vi "IOPanel_HandShake.vi"(11 "IOCard In":refnum<class "IOCard.lvclass">) -> ()   [LabVIEW 2019]
uses:
  Ctrl/IO Card_Type.ctl
  IO_Class/IOCard.lvclass
  <vilib>/Utility/miscctls.llb/LVPositionTypeDef.ctl
  IO_Class/IOCard.lvclass/IOCard.ctl
  LLB/Message/Ctrl/MsgDataInput.ctl
  LLB/Message/Ctrl/MsgPageSelect.ctl
  LLB/Message/Ctrl/LogType.ctl
  IO_Class/6480/6480.lvclass
  C:/Users/MyUser/Desktop/204J1_20201007/System/Function/IO Folder/IO_Class/IOCard.lvclass
  IO_Class/2410C/2410C-64.lvclass
  IO_Class/Zan/ZanCard.lvclass
  IO_Class/DMC1000B/DMC1000B.lvclass
  IO_Class/16InOut/16InOut.lvclass
  global/InAndOutGB.vi
  LLB/Commonly VI/Main Glb.vi
  <vilib>/Utility/config.llb/Read Key (String).vi
  LLB/Commonly VI.lvlib
  <vilib>/Utility/config.llb/NI_LVConfig.lvlib
  LLB/Message/MsgShowAndLog.lvlib
panel:
  out "IOCard":refnum<class "IOCard.lvclass">
  out "Card_Type":T1
  out "QName":string
  in  "Tab Control":enum32{"Input", "Output"}(tab)
  in  "Reconnect":bool
  out "Lst_Input":i32[](listbox) caption="Input"
  in  "Lst_Output":i32[](listbox)=[2] caption="Output"
  out "CardNumber":i32
  out "IOType":enum16{"Input", "Output"}(ring)=enum."Output"
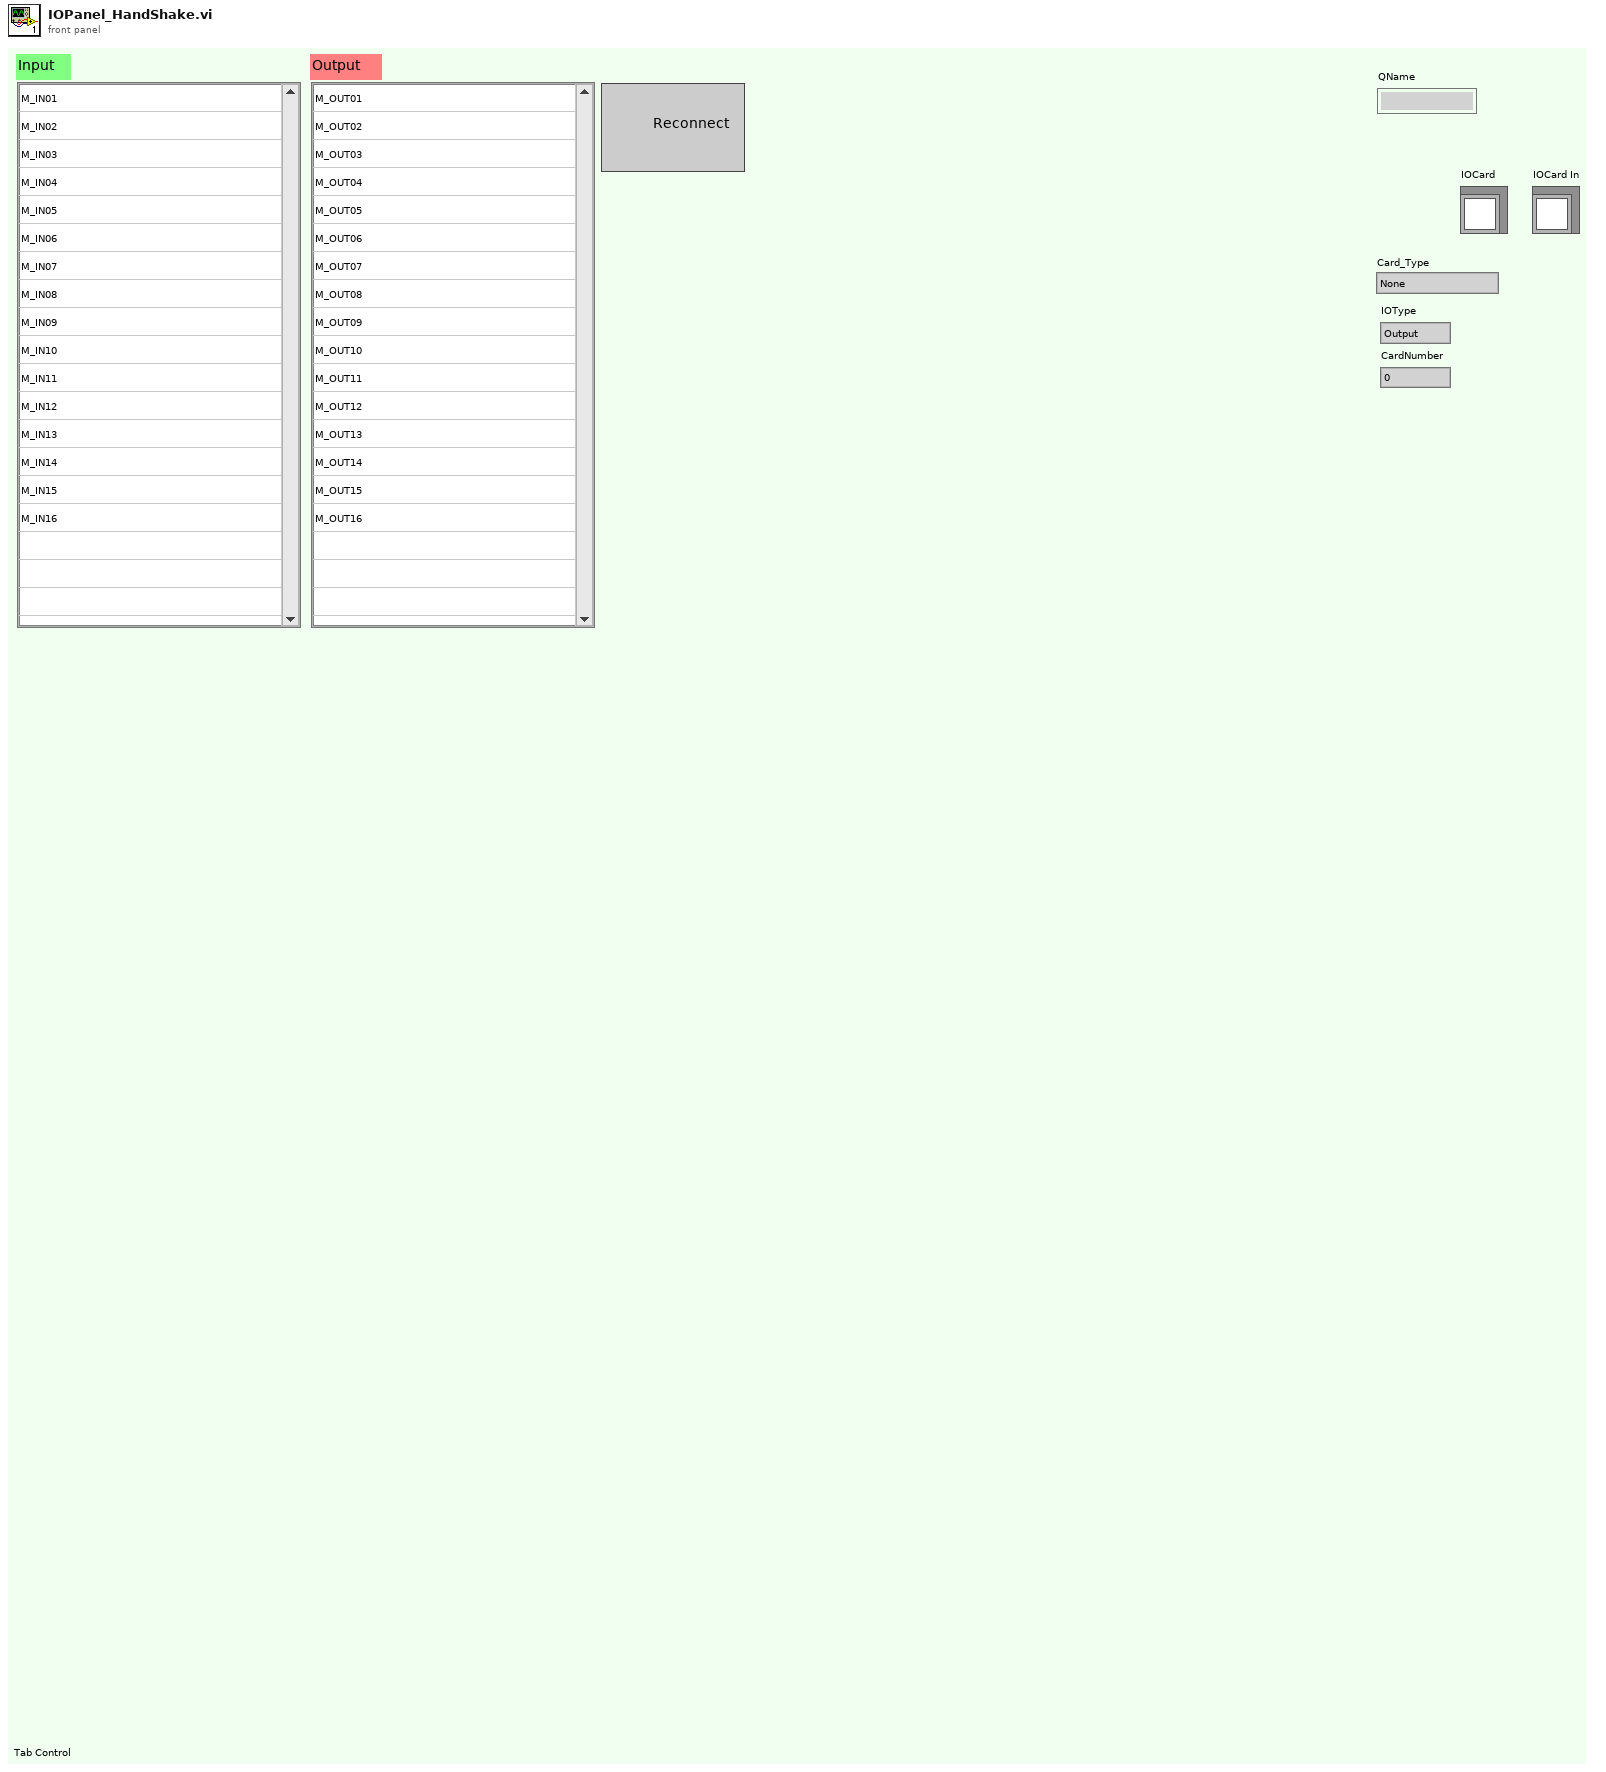
[diagram p1: front panel]
types:
  T1 = typedef "IO Card_Type.ctl" = enum16{"None", "Unidaq32", "6480", "2410C-64", "Zan", "DMC1000B", "16InOut", "Robot", "DMC3600"}
  T2 = typedef "LVPositionTypeDef.ctl" = cluster{"Left":i32, "Top":i32}
  T3 = cluster{"IO Card Type":T1, "IOType":enum16{"Input", "Output"}, "CardNumber":i32, "ConnectAct":bool, "IP":string}
  T4 = cluster{"CardNumber":i32, "Connect":bool, "Handler":i32}
  T5 = typedef "MsgDataInput.ctl" = cluster{"MsgPageSelect":T6, "LogType":T7, "Msg":string, "Time":string}
  T6 = typedef "MsgShowAndLog.lvlib/MsgPageSelect.ctl" = enum16{"System", "Comm", "IO", "Action", "Alarm"}
  T7 = typedef "MsgShowAndLog.lvlib/LogType.ctl" = enum16{"Auto", "Manual", "Handshake", "Error"}
  T8 = typedef "LVBoundsTypeDef.ctl" = cluster{"Width":u32, "Height":u32}
  T9 = typedef "LVPoint32TypeDef.ctl" = cluster{"Horizontal":i32, "Vertical":i32}
  T10 = typedef "NI_LVConfig.lvlib/Config Data RefNum.ctl" = refnum<k1>
  T11 = cluster{"Card":i32, "Connect":bool, "Handler":i32}[]
  T12 = cluster{"Card":i32, "Connect":bool, "Handler":i32}
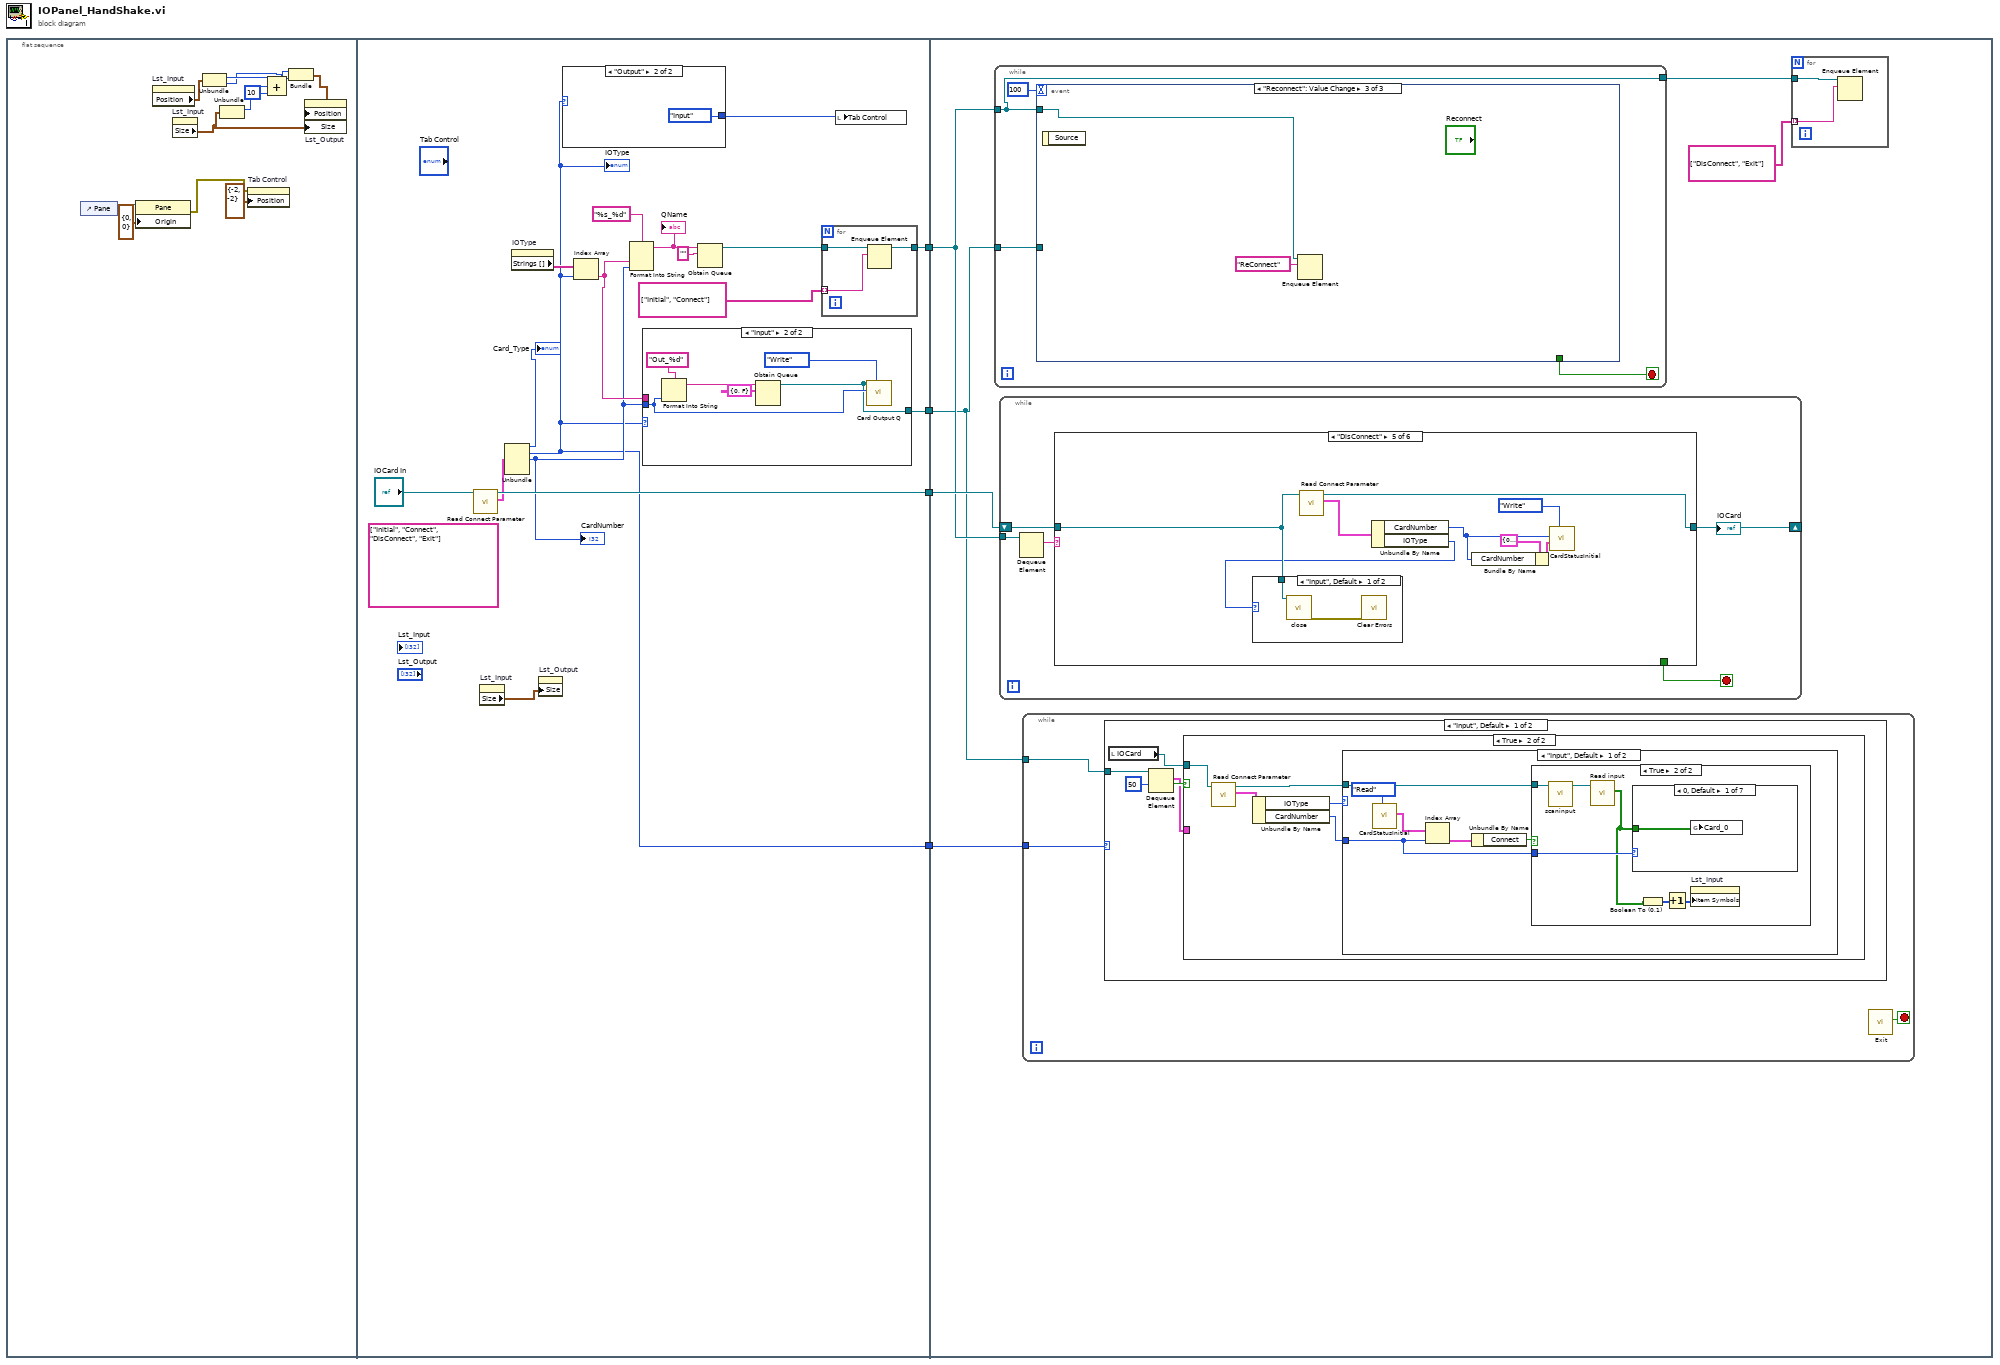
[diagram p0: block diagram]
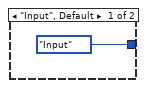
[diagram p2: hidden frame]
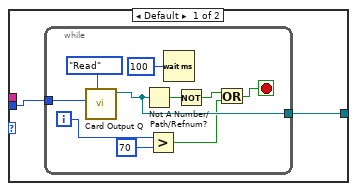
[diagram p3: hidden frame]
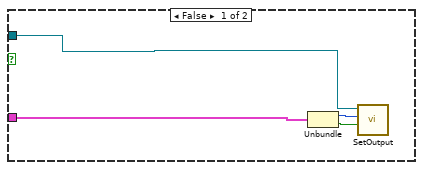
[diagram p4: hidden frame]
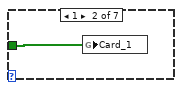
[diagram p6: hidden frame]
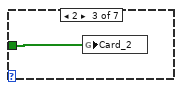
[diagram p7: hidden frame]
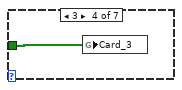
[diagram p8: hidden frame]
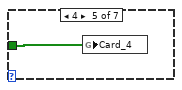
[diagram p9: hidden frame]
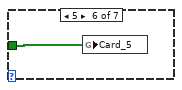
[diagram p10: hidden frame]
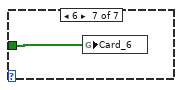
[diagram p11: hidden frame]
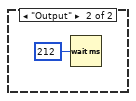
[diagram p13: hidden frame]
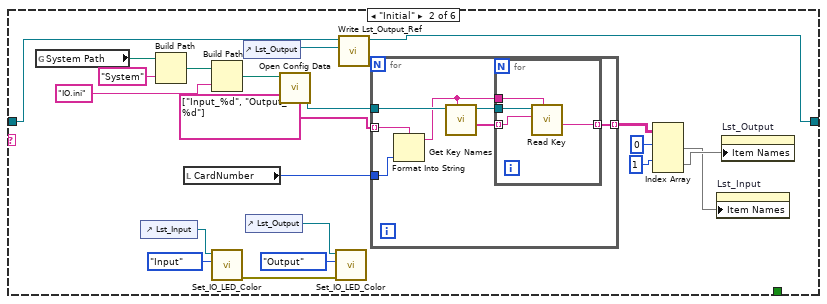
[diagram p15: hidden frame]
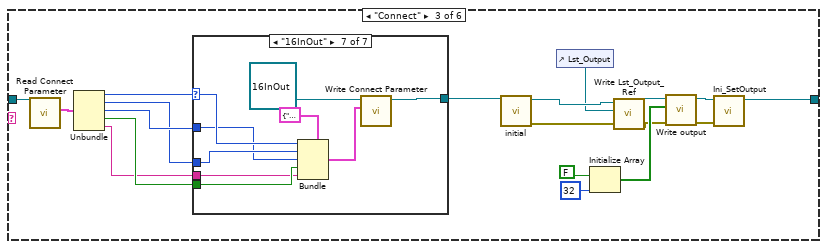
[diagram p16: hidden frame]
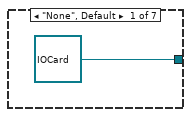
[diagram p17: hidden frame]
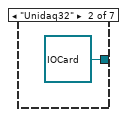
[diagram p18: hidden frame]
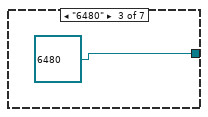
[diagram p19: hidden frame]
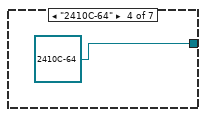
[diagram p20: hidden frame]
diagram:
  n1 = flat-sequence {
    tunnel: [w30] -> w4
    tunnel: [w25] -> w3
    tunnel: [w23] -> w2
    tunnel: [w17] -> w1
    tunnel: w4 -> [w62]
    tunnel: w3 -> [w59]
    tunnel: w2 -> [w58]
    tunnel: w1 -> [w57]
    frame #0 {
      n2 = control-ref of="Pane"() -> (w15:refnum<vi>)
      n3 = property class="Pane"(reference=w15, "Origin"=T2 {"Left"=0, "Top"=0} ("Position")) -> (error out=w13:errorcluster)  [unwired: 1 in, 1 out]
      n4 = property on="Lst_Input" class="LstBox (strict)"() -> ("Position"=w12:T2)  [unwired: 2 in, 2 out]
      n5 = property on="Lst_Input" class="LstBox (strict)"() -> ("Size"=w11:T8)  [unwired: 2 in, 2 out]
      n6 = Unbundle(w12) -> ("Left"=w10:i32, "Top"=w6:i32)
      n7 = Unbundle(w11) -> ("Width"=w9:u32)  [unwired: 1 out]
      n8 = property on="Tab Control" class="TabCtl (strict)"(error in=w13, "Position"=T2 {"Left"=-2, "Top"=-2}) -> ()  [unwired: 1 in, 2 out]
      n9 = Compound Arithmetic op=ADD(w10, w9, u32 10 ("value")) -> (w7:u32)
      n10 = Bundle(w7, "Top"=w6) -> (w5:cluster{u32, "Top":i32})  [unwired: 1 in]
      n11 = property on="Lst_Output" class="LstBox (strict)"("Position"=w5, "Size"=w11) -> ()  [unwired: 2 in, 2 out]
    }
    frame #1 {
      (unwired) string[] ["Initial", "Connect", "DisConnect", "Exit"]
      n12 = call "Read Connect Parameter.vi"("IOCard in"="IOCard In") -> ("Connect Parameter"=w29:T3, "IOCard out"=w30:refnum<class "IOCard.lvclass">)  [unwired: 8 in, 1 out]
      n13 = property on="Lst_Input" class="LstBox (strict)"() -> ("Size"=w18:T8)  [unwired: 2 in, 2 out]
      n14 = Unbundle(w29) -> ("IO Card Type"=→"Card_Type":T1, "IOType"=w17:enum16{"Input", "Output"}, "CardNumber"=w21:i32)  [unwired: 2 out]
      "CardNumber" <- w21
      "IOType" <- w17
      n15 = property on="IOType" class="Enum (strict)"() -> ("Strings []"=w28:string[])  [unwired: 2 in, 2 out]
      n16 = property on="Lst_Output" class="LstBox (strict)"("Size"=w18) -> ()  [unwired: 2 in, 2 out]
      n17 = case shown="\"Output\"" w17 {
        tunnel: [enum32{"Input", "Output"}."Input" ("Tab Control") enum32{"Input", "Output"}."Input" ("Tab Control")] -> w19
        frame "Input", Default {
        }
        frame "Output" {
        }
      }
      n18 = Index Array(array=w28, index=w17) -> (element=w24:string)
      n19 = Format Into String(format string="%s_%d", w24, w21) -> (resulting string=w32:string)  [unwired: 2 in, 1 out]
      "QName" <- w32
      n20 = case shown="\"Input\"" w17 {
        tunnel: w24 -> [_ _]
        tunnel: w21 -> [w37 w50]
        tunnel: [w36 w49] -> w23
        frame Default {
          n21 = while {
            tunnel: w37 -> [w46]
            tunnel: [w44] -> w36
            i -> [w40]
            stop <- w43 stop-if-true
            n22 = call "Card Output Q.vi"("Action"=enum16{"Initial", "Write", "Read", "Release"}."Read", "CardIndex"=w46) -> ("Output Q Out"=w44:refnum<queue>)  [unwired: 8 in, 1 out]
            n23 = Not A Number/Path/Refnum?(number/path/refnum=w44) -> (NaN/Path/Refnum?=w42:bool)
            n24 = Greater?(x=w40, y=70) -> (0:w39:bool)
            n25 = Wait (ms)(milliseconds to wait=u32 100) -> ()  [unwired: 1 out]
            n26 = Not(x=w42) -> (.not. x?=w41:bool)
            n27 = Or(x=w41, y=w39) -> (x .or. y?=w43:bool)
          }
        }
        frame "Input" {
          n28 = Format Into String(format string="Out_%d", w50) -> (resulting string=w48:string)  [unwired: 2 in, 1 out]
          n29 = Obtain Queue(name (unnamed)=w48, element data type=cluster{"Index":i32, "BL":bool} {"Index"=0, "BL"=FALSE}) -> (queue out=w49:refnum<queue>)  [unwired: 3 in, 2 out]
          n30 = call "Card Output Q.vi"("Action"=enum16{"Initial", "Write", "Read", "Release"}."Write", "CardIndex"=w50, "OutputQIn"=w49) -> ()  [unwired: 7 in, 2 out]
        }
      }
      n31 = Obtain Queue(name (unnamed)=w32, element data type="") -> (queue out=w26:refnum<queue>)  [unwired: 3 in, 2 out]
      n32 = for {
        tunnel: w26 -> [w56]
        tunnel: string[] ["Initial", "Connect"] -> [w55] mode=indexing
        tunnel: [w54] -> w25
        n33 = Enqueue Element(queue=w56, element=w55) -> (queue out=w54:refnum<queue>)  [unwired: 2 in, 2 out]
      }
      n34 = local write "Tab Control"(w19) -> ()
    }
    frame #2 {
      n35 = while {
        tunnel: w59 -> [w246]
        tunnel: [w246] -> w61
        tunnel: w58 -> [w245]
        stop <- w247 stop-if-true
        n36 = event shown="[2] \"Reconnect\": Value Change" {
          selector: _ -> [_ _ _]
          dyn-events: _ -> [_ _ _]
          timeout: 100 -> [_ _ _]
          tunnel: [w249 _ _] -> w247
          tunnel: w246 -> [_ _ w268]
          tunnel: w245 -> [_ w261 _]
          event Timeout {
            n37 = event-data() -> ()  [unwired: 1 in, 3 out]
            n38 = call "Exit.vi"() -> ("ExitOut"=w249:bool)  [unwired: 11 in]
          }
          event "Lst_Output": Double Click {
            n39 = event-data() -> ("CtlRef"=w266:refnum<vi>, "Coords"=w265:T9)  [unwired: 1 in, 1 out]
            n40 = invoke on="Invoke Node" class="LstBox (strict)" method="Point To Row"(reference=w266, "Point"=w265) -> (reference out=w262:refnum<vi>, "Row"=w253:i32)  [unwired: 5 in, 5 out]
            n41 = property on="Property Node" class="LstBox (strict)"(reference=w262) -> ("Item Symbols"=w250:i32[])  [unwired: 1 in, 2 out]
            n42 = Index Array(array=w250, index=w253) -> (element=w264:i32)
            n43 = Equal?(x=w264, y=1) -> (x = y?=w252:bool)
            n44 = Bundle(cluster=cluster{"Index":i32, "BL":bool} {"Index"=0, "BL"=FALSE} ("element"), "Index"=w253, "BL"=w252) -> (w260:cluster{"Index":i32, "BL":bool})
            n45 = local read "QName"() -> (w254:string)
            n46 = Enqueue Element(queue=w261, element=w260) -> (error out=w251:errorcluster)  [unwired: 2 in, 2 out]
            n47 = Format Into String(format string="%s,%d,%s", w254, w253, w252) -> (resulting string=w256:string)  [unwired: 2 in, 1 out]
            n48 = Bundle By Name(cluster=T5 {"MsgPageSelect"=enum."IO", "LogType"=enum."Manual", "Msg"="", "Time"=""} ("DataIn"), "Msg"=w256) -> (w258:T5)
            n49 = call "SendMsg.vi"("error in (no error)"=w251, "DataIn"=w258) -> ()  [unwired: 9 in, 1 out]
          }
          event "Reconnect": Value Change {
            n50 = event-data() -> ()  [unwired: 1 in, 1 out]
            n51 = Enqueue Element(queue=w268, element="ReConnect") -> ()  [unwired: 2 in, 3 out]
          }
        }
      }
      n52 = while {
        tunnel: w59 -> [w106]
        shift-right: [w104] -> _
        shift-left: w62 -> [w103]
        stop <- w102 stop-if-true
        n53 = Dequeue Element(queue=w106) -> (element=w105:string)  [unwired: 2 in, 3 out]
        n54 = case shown="\"DisConnect\"" w105 {
          tunnel: [w107 w116 w153 w194 w234 w243] -> w104
          tunnel: w103 -> [w107 w117 w158 w199 w235 w243]
          tunnel: [_ _ _ _ _ TRUE] -> w102
          frame "False", Default {
          }
          frame "Initial" {
            n55 = global read "Main Glb.vi" "System Path"() -> (w128:path)
            n56 = control-ref of="Lst_Input"() -> (w121:refnum<vi>)
            n57 = Build Path(base path=w128, name or relative path="System") -> (appended path=w126:path)
            n58 = local read "CardNumber"() -> (w108:i32)
            n59 = Build Path(base path=w126, name or relative path="IO.ini") -> (appended path=w124:path)
            n60 = call "Set_IO_LED_Color.vi"("SelectType"=enum16{"Input", "Output"}."Input", "ListBox Ref"=w121) -> ("error out"=w118:errorcluster)  [unwired: 9 in]
            n61 = control-ref of="Lst_Output"() -> (w115:refnum<vi>)
            n62 = control-ref of="Lst_Output"() -> (w122:refnum<vi>)
            n63 = call <vilib>:"Open Config Data.vi"("configuration file path"=w124) -> ("refnum"=w123:T10)  [unwired: 8 in, 2 out]
            n64 = call "Set_IO_LED_Color.vi"("error in (no error)"=w118, "SelectType"=enum16{"Input", "Output"}."Output", "ListBox Ref"=w122) -> ()  [unwired: 8 in, 1 out]
            n65 = call-dynamic "Write Lst_Output_Ref.vi"("Lst_Output_Ref"=w115, "IOCard in"=w117) -> ("IOCard out"=w116:refnum<class "IOCard.lvclass">)  [unwired: 8 in, 1 out]
            n66 = for {
              tunnel: w123 -> [w135]
              tunnel: [w132] -> w113 mode=indexing
              tunnel: string[] ["Input_%d", "Output_%d"] -> [w131] mode=indexing
              tunnel: w108 -> [w129]
              n67 = Format Into String(format string=w131, w129) -> (resulting string=w130:string)  [unwired: 2 in, 1 out]
              n68 = call <vilib>:"Get Key Names.vi"("section"=w130, "refnum"=w135) -> ("key names"=w133:string[], "refnum out"=w134:T10)  [unwired: 6 in, 2 out]
              n69 = for {
                tunnel: w134 -> [w139]
                tunnel: w133 -> [w138] mode=indexing
                tunnel: w130 -> [w137]
                tunnel: [w136] -> w132 mode=indexing
                n70 = call-poly <vilib>:"Read Key.vi"("section"=w137, "key"=w138, "refnum"=w139) -> ("value"=w136:string)  [unwired: 5 in, 3 out]
              }
            }
            n71 = Index Array(array=w113, index (row) #1=0 ("index (row)"), index (row) #2=1 ("index (row)")) -> (element #1=w109:string[], element #2=w110:string[])  [unwired: 2 in]
            n72 = property on="Lst_Input" class="LstBox (strict)"("Item Names"=w109) -> ()  [unwired: 2 in, 2 out]
            n73 = property on="Lst_Output" class="LstBox (strict)"("Item Names"=w110) -> ()  [unwired: 2 in, 2 out]
          }
          frame "Connect" {
            n74 = call "Read Connect Parameter.vi"("IOCard in"=w158) -> ("Connect Parameter"=w157:T3)  [unwired: 8 in, 2 out]
            n75 = Unbundle(w157) -> ("IO Card Type"=w156:T1, "IOType"=w154:enum16{"Input", "Output"}, "CardNumber"=w155:i32, "ConnectAct"=w151:bool, "IP"=w150:string)
            n76 = case shown="\"16InOut\"" w156 {
              selector: w156 -> [_ _ _ _ _ w169 w178]
              tunnel: [refnum<class "IOCard.lvclass"> refnum ("IOCard.lvclass") refnum<class "IOCard.lvclass"> refnum ("IOCard.lvclass") refnum<class "6480.lvclass"> refnum ("6480.lvclass") refnum<class "2410C-64.lvclass"> refnum ("2410C-64.lvclass") refnum<class "ZanCard.lvclass"> refnum ("ZanCard.lvclass") w172 w181] -> w149
              tunnel: w155 -> [_ _ _ _ _ w167 w176]
              tunnel: w154 -> [_ _ _ _ _ w168 w177]
              tunnel: w151 -> [_ _ _ _ _ w166 w175]
              tunnel: w150 -> [_ _ _ _ _ w165 w174]
              frame "None", Default {
              }
              frame "Unidaq32" {
              }
              frame "6480" {
              }
              frame "2410C-64" {
              }
              frame "Zan" {
              }
              frame "DMC1000B" {
                w164 = refnum<class "DMC1000B.lvclass"> refnum  # DMC1000B.lvclass
                n77 = Bundle(cluster=T3 {"IO Card Type"=enum."None", "IOType"=enum."Output", "CardNumber"=0, "ConnectAct"=FALSE, "IP"=""} ("Connect Parameter"), "IO Card Type"=w169, "IOType"=w168, "CardNumber"=w167, "ConnectAct"=w166, "IP"=w165) -> (w170:T3)
                n78 = call "Write Connect Parameter.vi"("Connect Parameter"=w170, "IOCard in"=w164) -> ("IOCard out"=w172:refnum<class "DMC1000B.lvclass">)  [unwired: 8 in, 1 out]
              }
              frame "16InOut" {
                n79 = Bundle(cluster=T3 {"IO Card Type"=enum."None", "IOType"=enum."Output", "CardNumber"=0, "ConnectAct"=FALSE, "IP"=""} ("Connect Parameter"), "IO Card Type"=w178, "IOType"=w177, "CardNumber"=w176, "ConnectAct"=w175, "IP"=w174) -> (w179:T3)
                n80 = call "Write Connect Parameter.vi"("Connect Parameter"=w179, "IOCard in"=refnum<class "16InOut.lvclass"> refnum ("16InOut.lvclass")) -> ("IOCard out"=w181:refnum<class "16InOut.lvclass">)  [unwired: 8 in, 1 out]
              }
            }
            n81 = call-dynamic "initial.vi"("IOCard in"=w149) -> ("error out"=w141:errorcluster, "IOCard out"=w152:refnum<class "IOCard.lvclass">)  [unwired: 9 in]
            n82 = control-ref of="Lst_Output"() -> (w142:refnum<vi>)
            n83 = Initialize Array(FALSE, 32 ("dimension size")) -> (w147:bool[])
            n84 = call-dynamic "Write Lst_Output_Ref.vi"("error in (no error)"=w141, "Lst_Output_Ref"=w142, "IOCard in"=w152) -> ("error out"=w144:errorcluster, "IOCard out"=w143:refnum<class "IOCard.lvclass">)  [unwired: 7 in]
            n85 = call-dynamic "Write output.vi"("error in (no error)"=w144, "output"=w147, "IOCard in"=w143) -> ("error out"=w140:errorcluster, "IOCard out"=w148:refnum<class "IOCard.lvclass">)  [unwired: 7 in]
            n86 = call-dynamic "Ini_SetOutput.vi"("error in (no error)"=w140, "IOCard in"=w148) -> ("IOCard out"=w153:refnum<class "IOCard.lvclass">)  [unwired: 8 in, 1 out]
          }
          frame "ReConnect" {
            n87 = call "Read Connect Parameter.vi"("IOCard in"=w199) -> ("Connect Parameter"=w198:T3)  [unwired: 8 in, 2 out]
            n88 = Unbundle(w198) -> ("IO Card Type"=w197:T1, "IOType"=w195:enum16{"Input", "Output"}, "CardNumber"=w196:i32, "ConnectAct"=w192:bool, "IP"=w191:string)
            n89 = case shown="\"16InOut\"" w197 {
              selector: w197 -> [_ _ _ _ _ w217 w229]
              tunnel: [refnum<class "IOCard.lvclass"> refnum ("IOCard.lvclass") refnum<class "IOCard.lvclass"> refnum ("IOCard.lvclass") refnum<class "6480.lvclass"> refnum ("6480.lvclass") refnum<class "2410C-64.lvclass"> refnum ("2410C-64.lvclass") refnum<class "ZanCard.lvclass"> refnum ("ZanCard.lvclass") w220 w232] -> w190
              tunnel: w196 -> [_ _ _ _ _ w215 w227]
              tunnel: w195 -> [_ _ _ _ _ w216 w228]
              tunnel: w192 -> [_ _ _ _ _ w214 w226]
              tunnel: w191 -> [_ _ _ _ _ w213 _]
              tunnel: "$VISA resource name" ("element") -> [_ _ _ _ _ _ w221]
              frame "None", Default {
              }
              frame "Unidaq32" {
              }
              frame "6480" {
              }
              frame "2410C-64" {
              }
              frame "Zan" {
              }
              frame "DMC1000B" {
                w212 = refnum<class "DMC1000B.lvclass"> refnum  # DMC1000B.lvclass
                n90 = Bundle(cluster=T3 {"IO Card Type"=enum."None", "IOType"=enum."Output", "CardNumber"=0, "ConnectAct"=FALSE, "IP"=""} ("Connect Parameter"), "IO Card Type"=w217, "IOType"=w216, "CardNumber"=w215, "ConnectAct"=w214, "IP"=w213) -> (w218:T3)
                n91 = call "Write Connect Parameter.vi"("Connect Parameter"=w218, "IOCard in"=w212) -> ("IOCard out"=w220:refnum<class "DMC1000B.lvclass">)  [unwired: 8 in, 1 out]
              }
              frame "16InOut" {
                n92 = call "SystemSearchDataName.vi"("element"=w221) -> ("variant"=w224:variant)  [unwired: 8 in, 2 out]
                n93 = Variant To Data(type=refnum<visa-resource-name> refnum ("VISA resource name"), Variant=w224) -> (data=w222:refnum<visa-resource-name>)  [unwired: 1 in, 1 out]
                n94 = Bundle(cluster=T3 {"IO Card Type"=enum."None", "IOType"=enum."Output", "CardNumber"=0, "ConnectAct"=FALSE, "IP"=""} ("Connect Parameter"), "IO Card Type"=w229, "IOType"=w228, "CardNumber"=w227, "ConnectAct"=w226, "IP"=w222) -> (w230:T3)
                n95 = call "Write Connect Parameter.vi"("Connect Parameter"=w230, "IOCard in"=refnum<class "16InOut.lvclass"> refnum ("16InOut.lvclass")) -> ("IOCard out"=w232:refnum<class "16InOut.lvclass">)  [unwired: 8 in, 1 out]
              }
            }
            n96 = call-dynamic "initial.vi"("IOCard in"=w190) -> ("error out"=w183:errorcluster, "IOCard out"=w193:refnum<class "IOCard.lvclass">)  [unwired: 9 in]
            n97 = control-ref of="Lst_Output"() -> (w184:refnum<vi>)
            n98 = Initialize Array(FALSE, 32 ("dimension size")) -> (w189:bool[])
            n99 = call-dynamic "Write Lst_Output_Ref.vi"("error in (no error)"=w183, "Lst_Output_Ref"=w184, "IOCard in"=w193) -> ("error out"=w186:errorcluster, "IOCard out"=w185:refnum<class "IOCard.lvclass">)  [unwired: 7 in]
            n100 = disable-structure shown="Enabled" {
              disable-tunnel: [w205 w206] -> w194
              disable-tunnel: w189 -> [w203 _]
              disable-tunnel: w186 -> [w202 _]
              disable-tunnel: w185 -> [w201 w206]
              frame Disabled {
                n101 = call-dynamic "Write output.vi"("error in (no error)"=w202, "output"=w203, "IOCard in"=w201) -> ("error out"=w200:errorcluster, "IOCard out"=w204:refnum<class "IOCard.lvclass">)  [unwired: 7 in]
                n102 = call-dynamic "Ini_SetOutput.vi"("error in (no error)"=w200, "IOCard in"=w204) -> ("IOCard out"=w205:refnum<class "IOCard.lvclass">)  [unwired: 8 in, 1 out]
              }
              frame Enabled {
              }
            }
          }
          frame "DisConnect" {
            n103 = call "Read Connect Parameter.vi"("IOCard in"=w235) -> ("Connect Parameter"=w239:T3, "IOCard out"=w234:refnum<class "IOCard.lvclass">)  [unwired: 8 in, 1 out]
            n104 = Unbundle By Name(w239) -> ("CardNumber"=w236:i32, "IOType"=w233:enum16{"Input", "Output"})
            n105 = case shown="\"Input\", Default" w233 {
              tunnel: w235 -> [w241 _]
              frame "Input", Default {
                n106 = call-dynamic "close.vi"("IOCard in"=w241) -> ("error out"=w242:errorcluster)  [unwired: 9 in, 1 out]
                n107 = call <vilib>:"Clear Errors.vi"("error in (no error)"=w242) -> ()  [unwired: 5 in, 2 out]
              }
              frame "Output" {
              }
            }
            n108 = Bundle By Name(cluster=T4 {"CardNumber"=0, "Connect"=FALSE, "Handler"=0} ("DataIn"), "CardNumber"=w236) -> (w237:T4)
            n109 = call "CardStatusInitial.vi"("Action"=enum16{"Initial", "Write", "Read", "Release"}."Write", "DataIn"=w237, "CardNumber"=w236) -> ()  [unwired: 8 in, 1 out]
          }
          frame "Exit" {
          }
        }
        "IOCard" <- w104
      }
      n110 = while {
        tunnel: w58 -> [w64]
        tunnel: w57 -> [w63]
        stop <- w65 stop-if-true
        n111 = case shown="\"Input\", Default" w63 {
          tunnel: w64 -> [w70 _]
          frame "Input", Default {
            n112 = local read "IOCard"() -> (w66:refnum<class "IOCard.lvclass">)
            n113 = Dequeue Element(queue=w70, timeout in ms (-1)=50) -> (element=w67:cluster{"Index":i32, "BL":bool}, timed out?=w68:bool)  [unwired: 1 in, 2 out]
            n114 = case shown="True" w68 {
              tunnel: w67 -> [w74 _]
              tunnel: w66 -> [w71 w77]
              frame False {
                n115 = Unbundle(w74) -> ("Index"=w73:i32, "BL"=w72:bool)
                n116 = call-dynamic "SetOutput.vi"("Boolean"=w72, "Index"=w73, "IOCard in"=w71) -> ()  [unwired: 6 in, 3 out]
              }
              frame True {
                n117 = call "Read Connect Parameter.vi"("IOCard in"=w77) -> ("Connect Parameter"=w76:T3, "IOCard out"=w78:refnum<class "IOCard.lvclass">)  [unwired: 8 in, 1 out]
                n118 = Unbundle By Name(w76) -> ("IOType"=w75:enum16{"Input", "Output"}, "CardNumber"=w79:i32)
                n119 = case shown="\"Input\", Default" w75 {
                  tunnel: w78 -> [w85 _]
                  tunnel: w79 -> [w80 _]
                  frame "Input", Default {
                    n120 = call "CardStatusInitial.vi"("Action"=enum16{"Initial", "Write", "Read", "Release"}."Read") -> ("CardStatus"=w83:T11)  [unwired: 10 in]
                    n121 = Index Array(array=w83, index=w80) -> (element=w82:T12)
                    n122 = Unbundle By Name(w82) -> ("Connect"=w81:bool)
                    n123 = case shown="True" w81 {
                      tunnel: w85 -> [_ w90]
                      tunnel: w80 -> [_ w89]
                      frame False {
                      }
                      frame True {
                        n124 = call-dynamic "scaninput.vi"("IOCard in"=w90) -> ("IOCard out"=w91:refnum<class "IOCard.lvclass">)  [unwired: 9 in, 1 out]
                        n125 = call-dynamic "Read input.vi"("IOCard in"=w91) -> ("input"=w88:bool[])  [unwired: 8 in, 2 out]
                        n126 = case shown="0, Default" w89 {
                          tunnel: w88 -> [w92 w93 w94 w95 w96 w97 w98]
                          frame 0, Default {
                            n127 = global write "InAndOutGB.vi" "Card_0"(w92) -> ()
                          }
                          frame 1 {
                            n128 = global write "InAndOutGB.vi" "Card_1"(w93) -> ()
                          }
                          frame 2 {
                            n129 = global write "InAndOutGB.vi" "Card_2"(w94) -> ()
                          }
                          frame 3 {
                            n130 = global write "InAndOutGB.vi" "Card_3"(w95) -> ()
                          }
                          frame 4 {
                            n131 = global write "InAndOutGB.vi" "Card_4"(w96) -> ()
                          }
                          frame 5 {
                            n132 = global write "InAndOutGB.vi" "Card_5"(w97) -> ()
                          }
                          frame 6 {
                            n133 = global write "InAndOutGB.vi" "Card_6"(w98) -> ()
                          }
                        }
                        n134 = Boolean To (0,1)(Boolean=w88) -> (0, 1=w87:i16[])
                        n135 = Increment(x=w87) -> (x+1=w86:i16[])
                        n136 = property on="Lst_Input" class="LstBox (strict)"("Item Symbols"=w86) -> ()  [unwired: 2 in, 2 out]
                      }
                    }
                  }
                  frame "Output" {
                  }
                }
              }
            }
          }
          frame "Output" {
            n137 = Wait (ms)(milliseconds to wait=u32 212) -> ()  [unwired: 1 out]
          }
        }
        n138 = call "Exit.vi"() -> ("ExitOut"=w65:bool)  [unwired: 11 in]
      }
      n139 = for {
        tunnel: w61 -> [w101]
        tunnel: string[] ["DisConnect", "Exit"] -> [w100] mode=indexing
        n140 = Enqueue Element(queue=w101, element=w100) -> ()  [unwired: 2 in, 3 out]
      }
    }
  }
